vi "aal_DZT (real input).vi"(0 "x":dbl[](array[numeric]), 1 "M":i32, 2 "index":i32, 3 "out_len":i32, 4 "fft_len":i32) -> (5 "Y":cdb[](array[numeric]), 6 "error":i32)   [LabVIEW 2017, in "NI_AALPro.lvlib"]
doc: "This function returns portion of single side band FFT of a real input signal.\n\nInputs:\n\n M : zoom in factor\n x : real input signal, with length of x_len\n index : initial index of the signal side band FFT where the \"zoom-in\" FFT starts.\n\noutputs:\n Y : output of the \"zoom in\" FFT with length of x_len/M/2. .\n\nSome restrictions applied on the input parameters:\n1. Signal length (x_len) must be mutiple of zoom in factor M.\n2. index >= 0, and (index+x_len/M/2)<x_len/2."
uses:
  NI_AALPro.lvlib
  lvanlys.dll
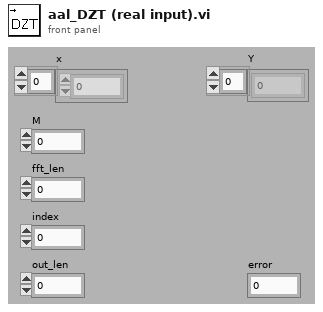
[diagram p1: front panel]
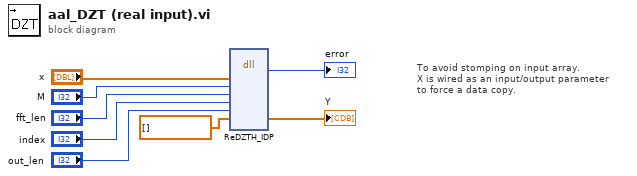
[diagram p0: block diagram]
diagram:
  # "To avoid stomping on input array.  \nX is wired as an input/output parameter \nto force a data copy."
  n1 = dll-call lib="C:/Program Files/National Instruments/LabVIEW 2017/resource/lvanlys.*" fn="ReDZTH_IDP"("x"="x", "M"="M", "fft_len"="fft_len", "index"="index", "out_len"="out_len", "y"=cdb[] [] ("Y")) -> ("return type"=→"error":i32, "y"=→"Y":cdb[])  [unwired: 10 in, 2 out]
